vi "AI config UI to not UI.vi"(10 "input terminal configuration":i32(ring)=-1 items=["Default"=-1, "RSE"=10083, "NRSE"=10078, "Differential"=10106, "Pseudodifferential"=12529], 11 "AI Config (UI)":T1 {"AI.Coupling" items=["AC"=10045, "DC"=10050, "GND"=10066]}) -> (3 "AI Config":T5 {"input terminal configuration" items=["default"=-1, "RSE"=10083, "NRSE"=10078, "Differential"=10106, "Pseudodifferential"=12529]; "AI.Coupling" items=["AC"=10045, "DC"=10050, "GND"=10066]})   [LabVIEW 2016, in "Instrument.Lockin.lvclass"]
uses:
  Instrument.Lockin.lvclass
  LockinDAQ/Typedefs/AI.coupling-enum.ctl
  LockinDAQ/LockinDAQ.lvclass
  LockinDAQ/Typedefs/446xAI-enum.ctl
  LockinDAQ/Typedefs/DAQType-enum.ctl
  LockinDAQ/Typedefs/AI.config-cluster.ctl
  LockinDAQ/Typedefs/AI.config(UI)-cluster.ctl
  LockinDAQ/Typedefs/AI.config(UI)-array.ctl
  LockinDAQ/Typedefs/AI.config-array.ctl
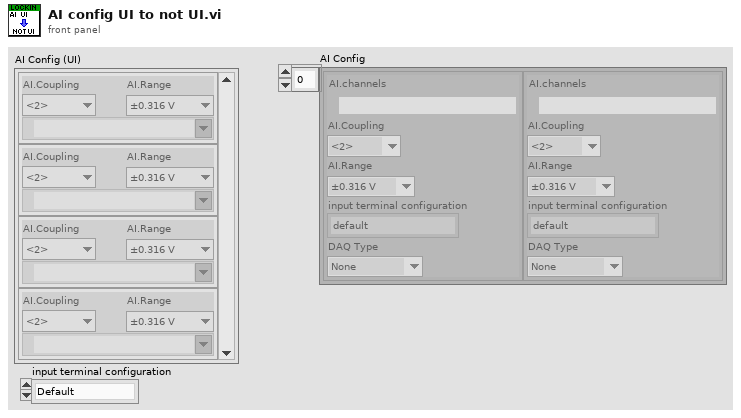
[diagram p1: front panel]
types:
  T1 = typedef "LockinDAQ.lvclass/AI.config(UI)-array.ctl" = T2[]
  T2 = typedef "LockinDAQ.lvclass/AI.config(UI)-cluster.ctl" = cluster{"AI.Coupling":T3, "AI.channels":tag, "AI.Range":T4}
  T3 = typedef "LockinDAQ.lvclass/AI.coupling-enum.ctl" = u16
  T4 = typedef "LockinDAQ.lvclass/446xAI-enum.ctl" = enum16{"±0.316 V", "±1.00 V", "±3.16 V", "±10.0 V", "±31.6 V", "±42.4 V"}
  T5 = typedef "LockinDAQ.lvclass/AI.config-array.ctl" = T6[]
  T6 = typedef "LockinDAQ.lvclass/AI.config-cluster.ctl" = cluster{"AI.channels":tag, "AI.Coupling":T3, "AI.Range":T4, "input terminal configuration":i32, "DAQ Type":T7}
  T7 = typedef "LockinDAQ.lvclass/DAQType-enum.ctl" = enum16{"None", "USB 4431", "PXI 446x"}
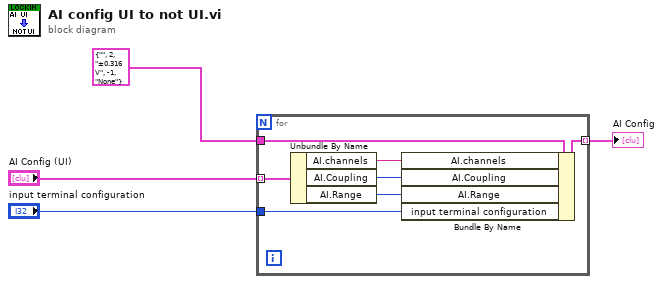
[diagram p0: block diagram]
diagram:
  n1 = for {
    tunnel: T6 {"AI.channels"="", "AI.Coupling"=2, "AI.Range"=enum."±0.316 V", "input terminal configuration"=-1, "DAQ Type"=enum."None"} ("AI.Config") -> [w11]
    tunnel: "AI Config (UI)" -> [w10] mode=indexing
    tunnel: [w5] -> w4 mode=indexing
    tunnel: "input terminal configuration" -> [w6]
    n2 = Unbundle By Name(w10) -> ("AI.channels"=w9:tag, "AI.Coupling"=w8:T3, "AI.Range"=w7:T4)
    n3 = Bundle By Name(cluster=w11, "AI.channels"=w9, "AI.Coupling"=w8, "AI.Range"=w7, "input terminal configuration"=w6) -> (w5:T6)
  }
  "AI Config" <- w4
